vi "Main.vi"() -> ()   [LabVIEW 2013]
doc: "This template is for the Queued Message Handler design pattern.\n\nThe Event Handling Loop generates messages based on user interface actions.\n\nThe Message Handling Loop processes messages generated by the Event Handling Loop, or by other messages. The messages are string values, so new messages can be added easily to the Message Cases case structure in the Message Handling Loop. Each message cluster can also provide an optional value for Message Data, which is a variant that can be converted to whatever message-specific data is required."
uses:
  <vilib>/vision/Image Controls.llb/IMAQ Image.ctl
  Message Passing/MsgQ Loops enum.ctl
  Image Processing/Mask ROI FG Enum.ctl
  System Status/Status FG Enum.ctl
  Globals/Average Sector Data.vi
  controls/UI Data.ctl
  Message Queue/Message Queue.lvlib
  User Event - Stop/User Event - Stop.lvlib
  Image Processing/Image Processing.lvlib
  Common/State Machines/State Machine Lib.lvlib
  Message Passing/Main MsgQ.lvlib
  Common/GUI/GUI.lvlib
  <vilib>/rvi/interface/nirviReadWriteControl/nirviReadWriteControl.xnode
  FGs/FPGA_Reference.ctl
  FPGA Bitfiles/8-Tap8-bitCamera_FPGATarget_8-Tap8-bit_Serial_Server.lvbitx
  <vilib>/rvi/errors/niLvFpgaMergeErrorWithErrorCode.vi
  NiFpgaLv.dll
  <vilib>/rvi/errors/niLvFpgaAdjustHostInterfaceError.vi
panel:
  out "Analysis Ticks":u32
  out "Accumulate Ticks":u32
  out "FPGA Display Image":T1(plugin-control)
  out "Right Wingbeat Avg Graph":u8[](graph)
  in  "Start Serial Server":bool=TRUE
  out "Left Wingbeat Avg Graph":u8[](graph)
  in  "Stop Charts":bool
  in  "Wing ROIs":T2
  out "FPGA image info":T5={"Image Type"=0, "Unit"=enum."Undefined", "X Resolution"=2040, "Y Resolution"=1088, "X Step"=1.0, "Y Step"=1.0, "Image Name"="Image"} {"Image Type" items=["Grayscale (U8)", "Grayscale (I16)", "Grayscale (SGL)", "Complex (CSG)", "RGB (U32)", "HSL (U32)", "RGB (U64)", "Grayscale (U16)"]}
  in  "Stream?":bool
  out "FPGA Image":T1
  in  "Test Visual Response":bool
  in  "Test FPGA":bool
  out "Status Update":string="VI Stopped"
  in  "Define Mask":bool
  in  "Acquire Image":bool
  in  "Stop":bool
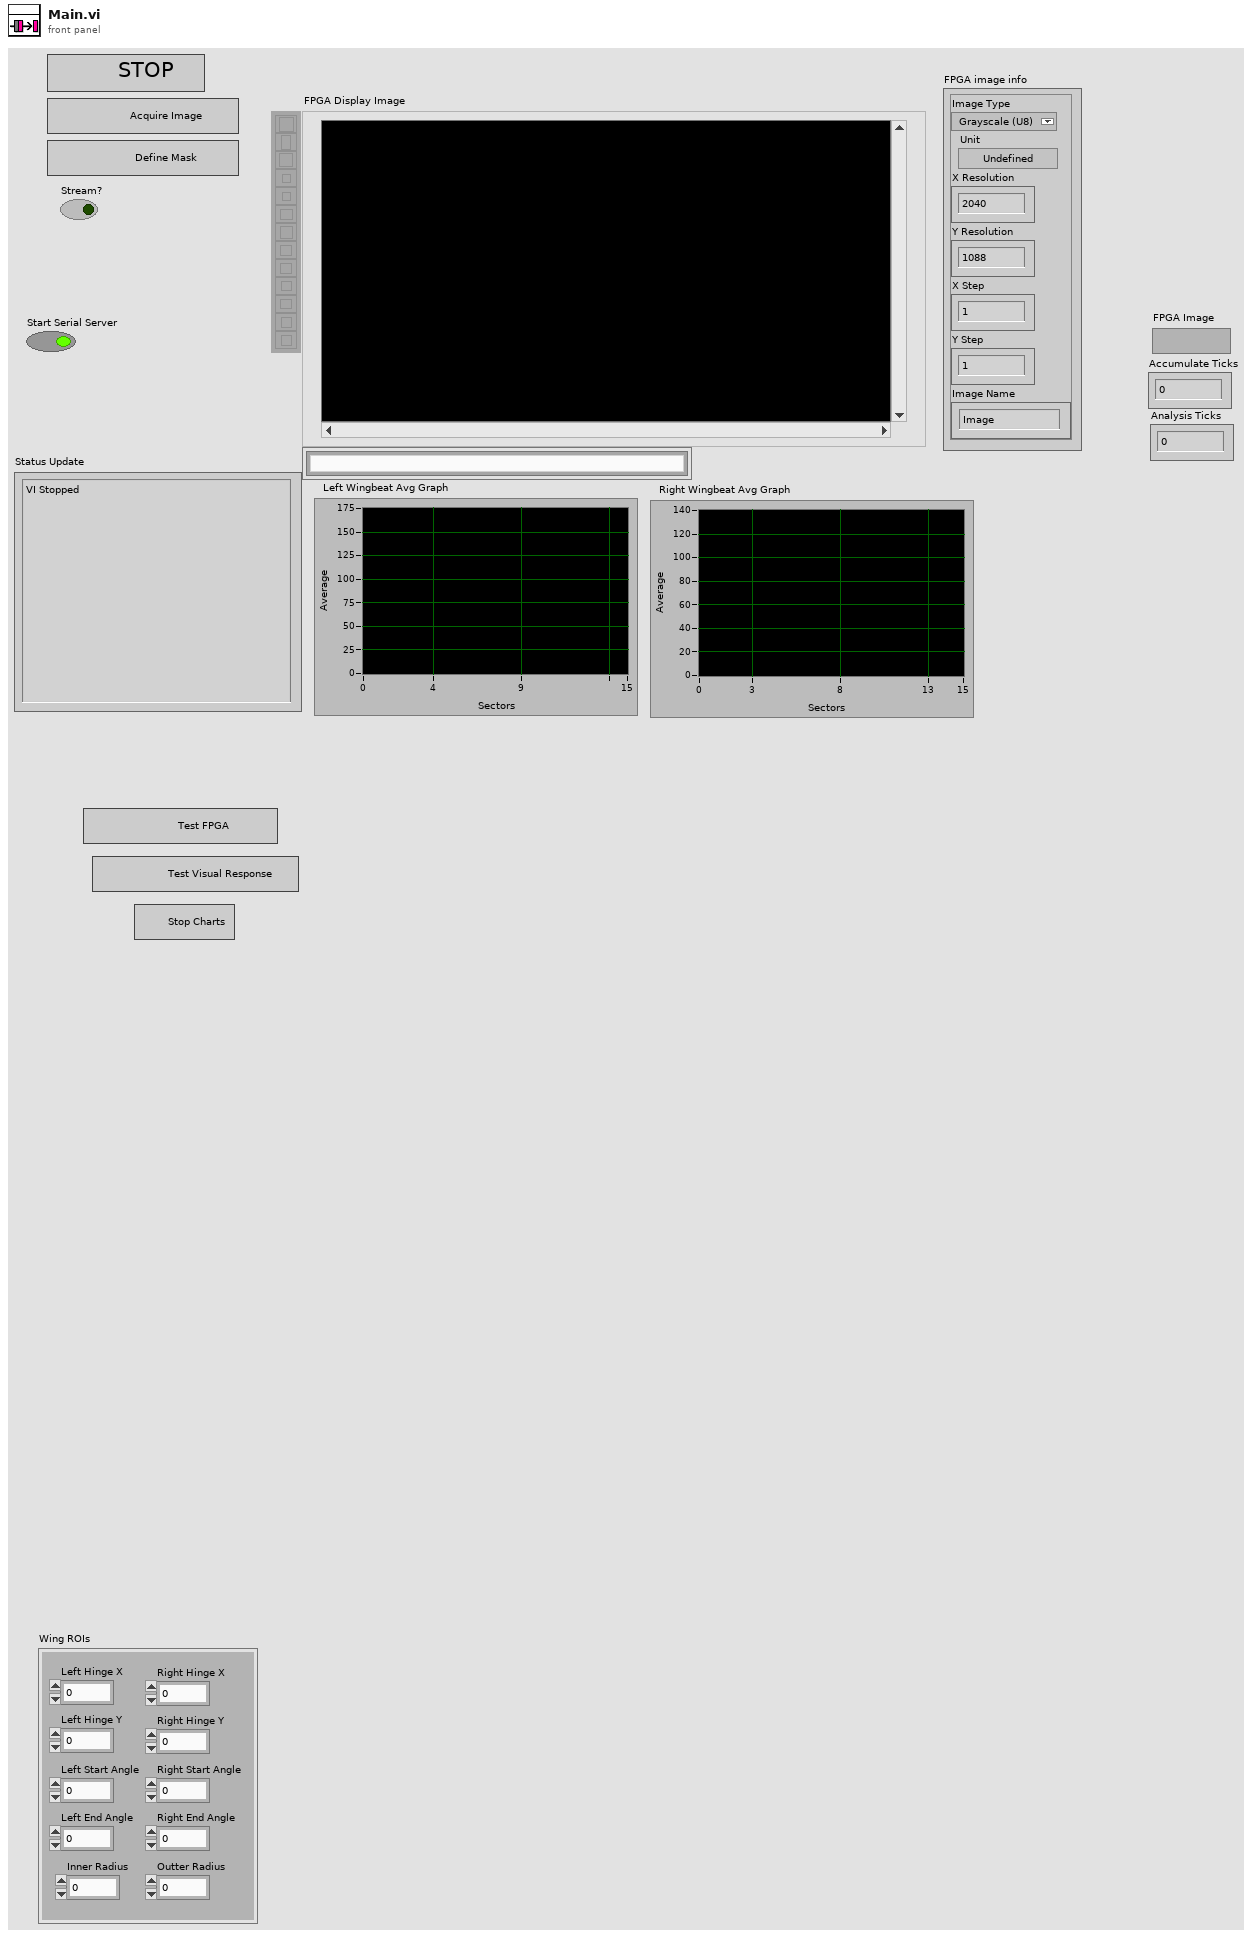
[diagram p1: front panel]
types:
  T1 = typedef "IMAQ Image.ctl" = refnum<image>
  T2 = cluster{"Left Hinge X":u16, "Left Hinge Y":u16, "Inner Radius":u16, "Outter Radius":u16, "Right Hinge X":u16, "Right Hinge Y":u16, "Right Start Angle":i16, "Right End Angle":i16, "Left Start Angle":i16, "Left End Angle":i16}
  T3 = typedef "Image Type" = u32
  T4 = typedef "Image Unit" = enum32{"Undefined", "Angström", "Micrometer", "Millimeter", "Centimeter", "Meter", "Kilometer", "Microinch", "Inch", "Feet", "Nautical miles", "Standard miles", "Steps"}
  T5 = cluster{"Image Type":T3, "Unit":T4, "X Resolution":i32, "Y Resolution":i32, "X Step":sgl, "Y Step":sgl, "Image Name":string}
  T6 = typedef "State Machine Lib.lvlib/STATE cluster.ctl" = cluster{"State":string, "Parameters":variant}
  T7 = typedef "Main MsgQ.lvlib/MsgQ Loops enum.ctl" = enum16{"User Interface", "Image Acq"}
  T8 = typedef "Status FG Enum.ctl" = enum16{"Reset", "Read", "Write"}
  T9 = typedef "Mask ROI FG Enum.ctl" = enum16{"Read", "Write"}
  T10 = typedef "FPGA_Reference.ctl" = refnum<k20>
  T11 = typedef "Mask ROI Cluster.ctl" = cluster{"left annulus":T12, "right annulus":T12, "Threshold Range":cluster{"Lower value":dbl, "Upper value":dbl}, "[Avg BG]":u8[], "Number of Sectors":u8, "Left ROI":T13, "Right ROI":T13, "Left Start Angle Duty Cycle":fxp<+,8,0>, "Left End Angle Duty Cycle":fxp<+,8,0>, "Right End Angle Duty Cycle":fxp<+,8,0>, "Right Start Angle Duty Cycle":fxp<+,8,0>, "[Sector ROIs]":T13[]}
  T12 = typedef "IMAQ Circle" = cluster{"Center X":i32, "Center Y":i32, "Inner Radius":i32, "Outer Radius":i32, "Start Angle":dbl, "End Angle":dbl}
  T13 = typedef "ROI Descriptor" = cluster{"Global Rectangle":i32[], "Contours":cluster{"ID":enum32{"External", "Internal"}, "Type":u32, "Coordinates":i32[]}[]}
  T14 = typedef "UI Data.ctl" = cluster{"Boolean <Replace Me>":bool, "Initial Message":string, "Numeric <Replace Me>":dbl, "Acquire Image Ref":refnum<vi>, "Define Mask Ref":refnum<vi>, "Status Update Ref":refnum<vi>, "Stop Button Ref":refnum<vi>, "FPGA Image":T1, "Processed Image":T1, "Left Annulus":cluster{"Center X":i32, "Center Y":i32, "Inner Radius":i32, "Outer Radius":i32, "Start Angle":dbl, "End Angle":dbl}, "Right Annulus":cluster{"Center X":i32, "Center Y":i32, "Inner Radius":i32, "Outer Radius":i32, "Start Angle":dbl, "End Angle":dbl}}
  T15 = typedef "Message Queue.lvlib/All Message Queues.ctl" = cluster{"UI":refnum<queue>}
  T16 = cluster{"Center X":i32, "Center Y":i32, "Inner Radius":i32, "Outer Radius":i32, "Start Angle":dbl, "End Angle":dbl}
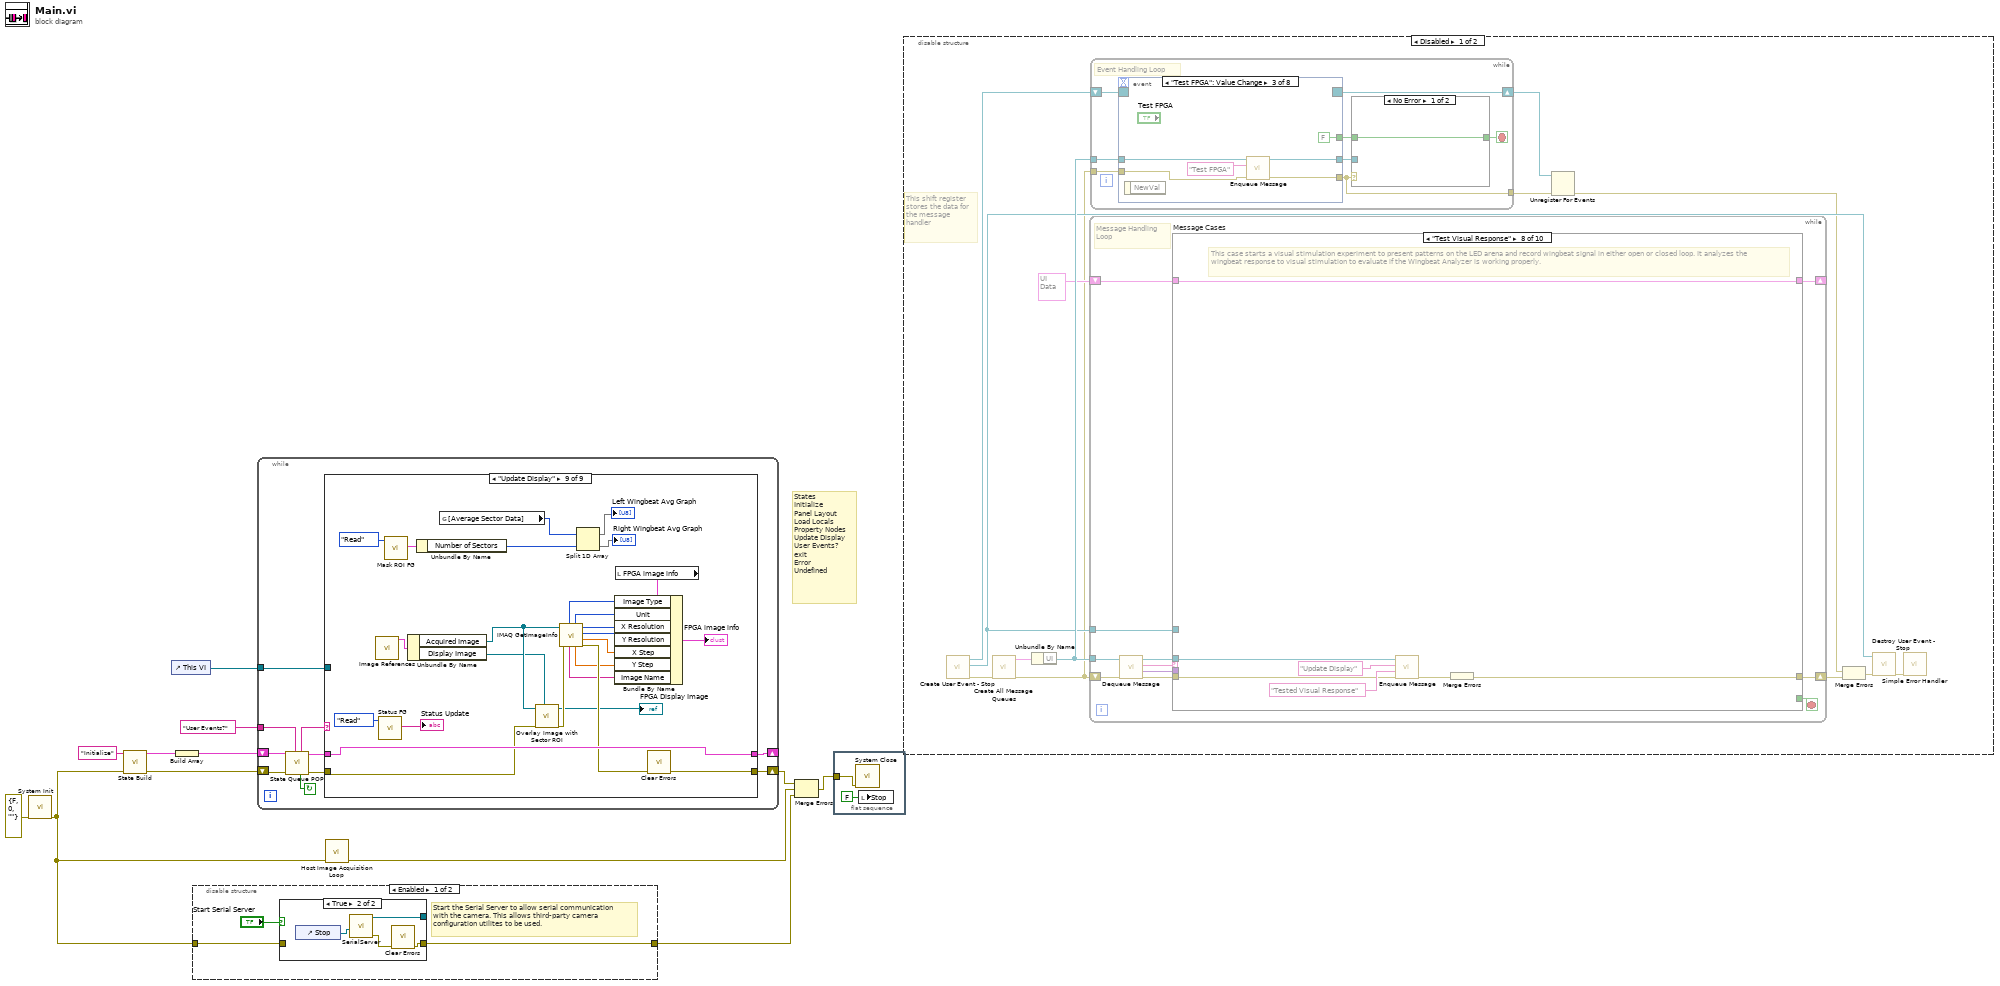
[diagram p0: block diagram]
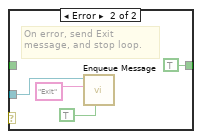
[diagram p4: hidden frame]
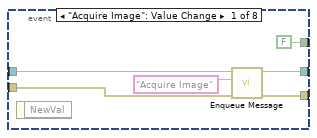
[diagram p5: hidden frame]
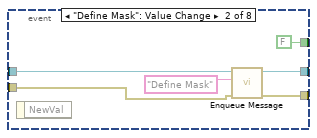
[diagram p6: hidden frame]
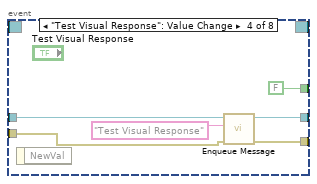
[diagram p7: hidden frame]
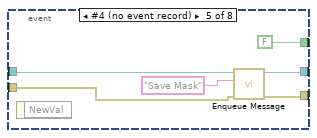
[diagram p8: hidden frame]
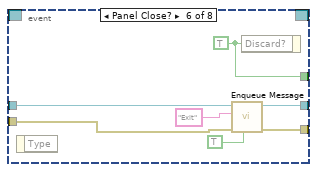
[diagram p9: hidden frame]
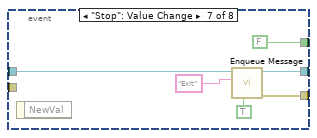
[diagram p10: hidden frame]
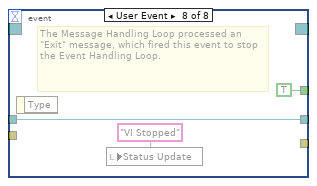
[diagram p11: hidden frame]
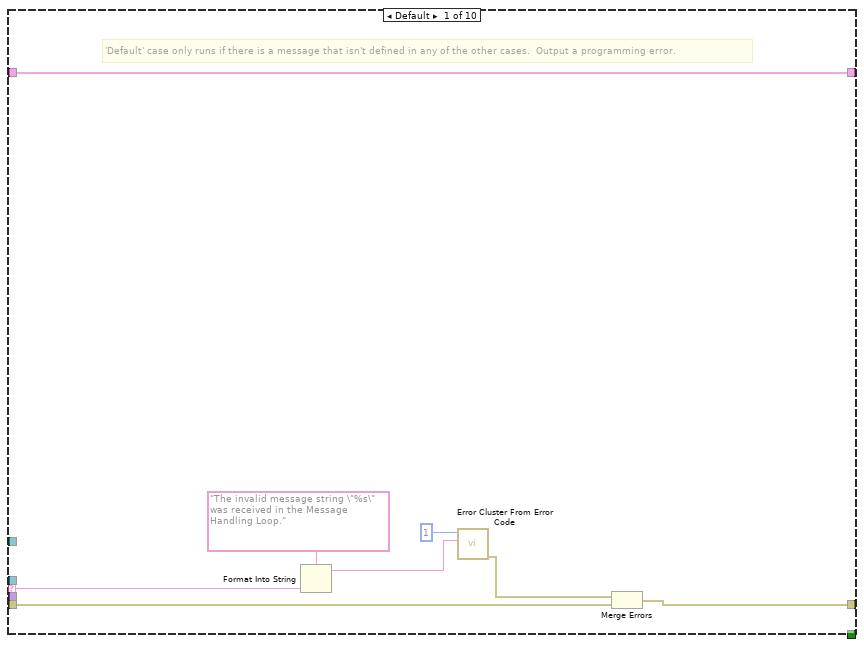
[diagram p12: hidden frame]
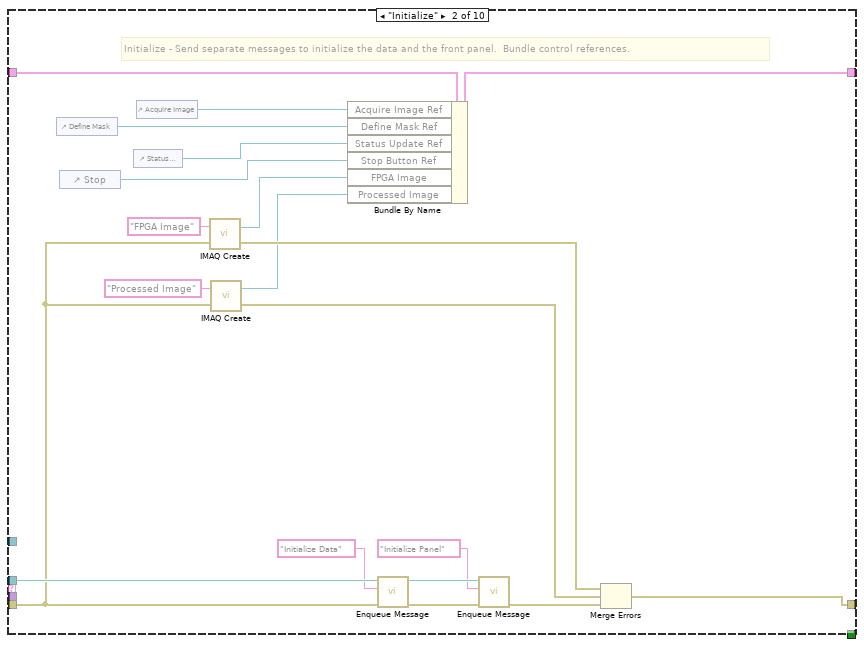
[diagram p13: hidden frame]
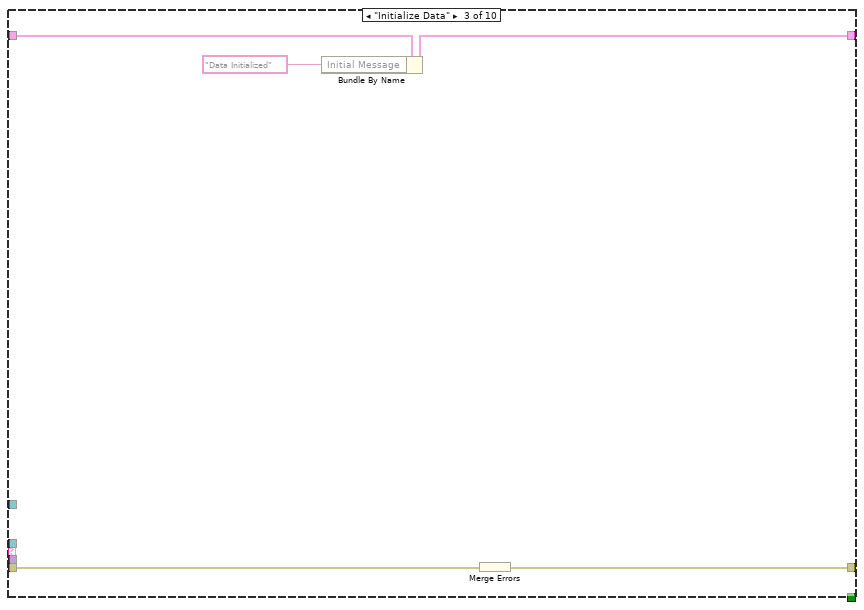
[diagram p14: hidden frame]
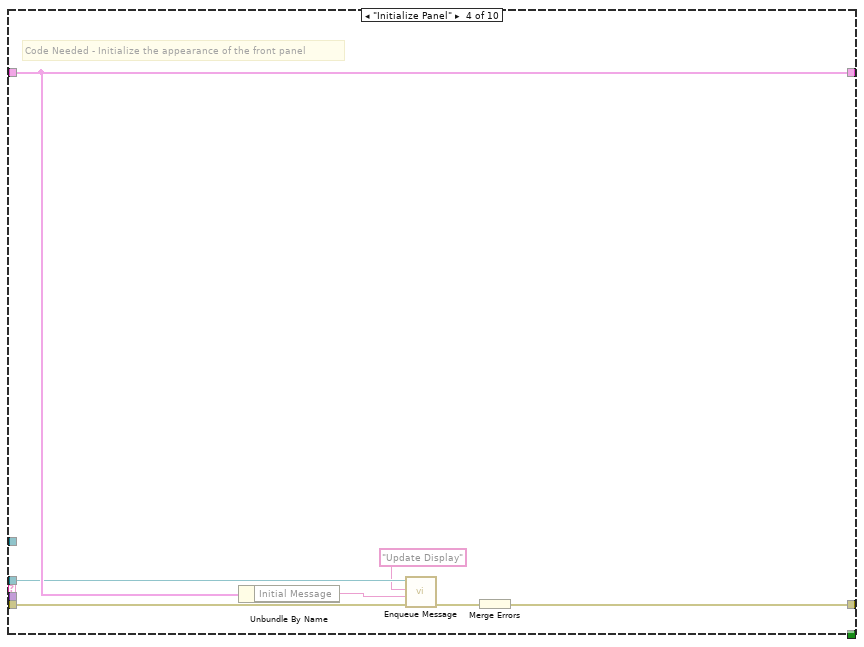
[diagram p15: hidden frame]
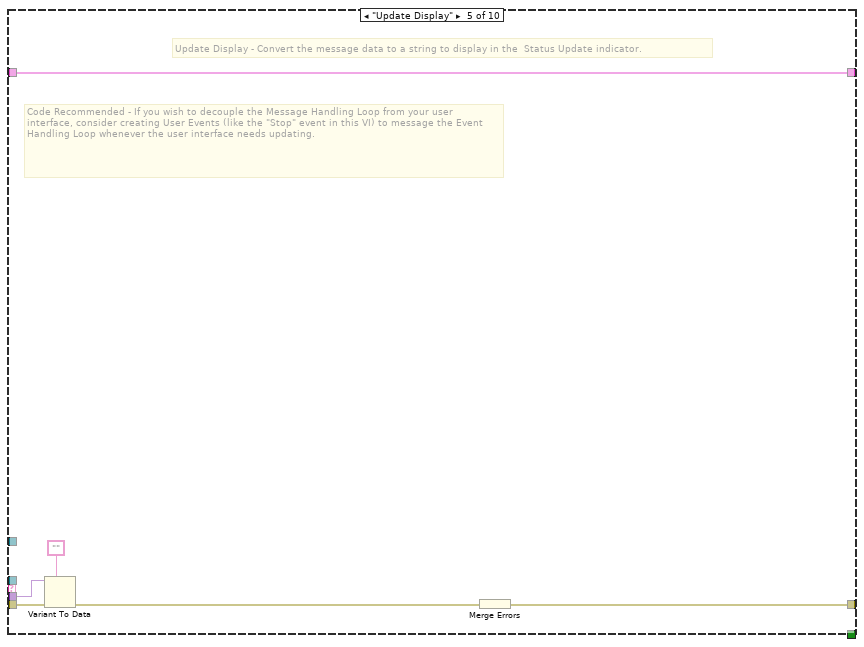
[diagram p16: hidden frame]
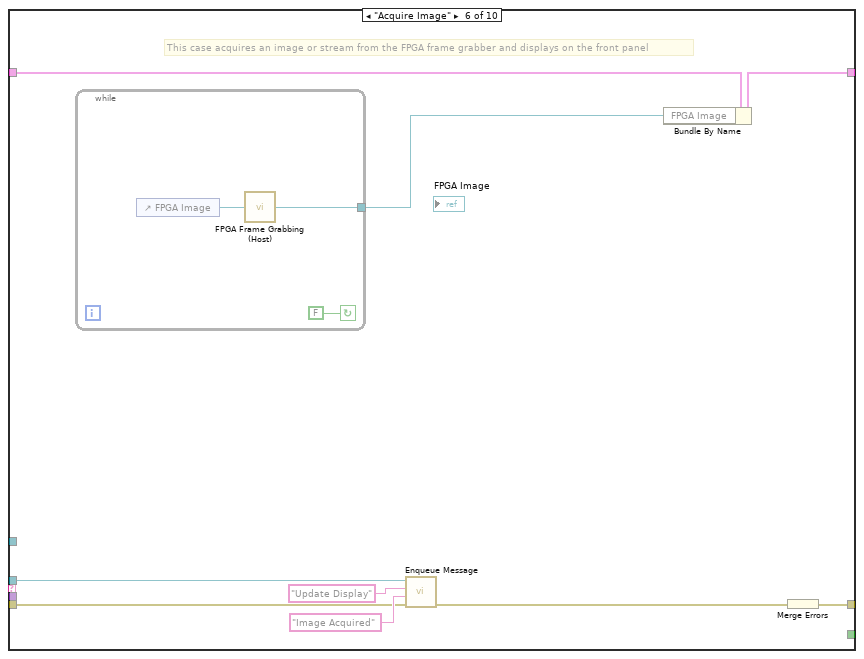
[diagram p17: hidden frame]
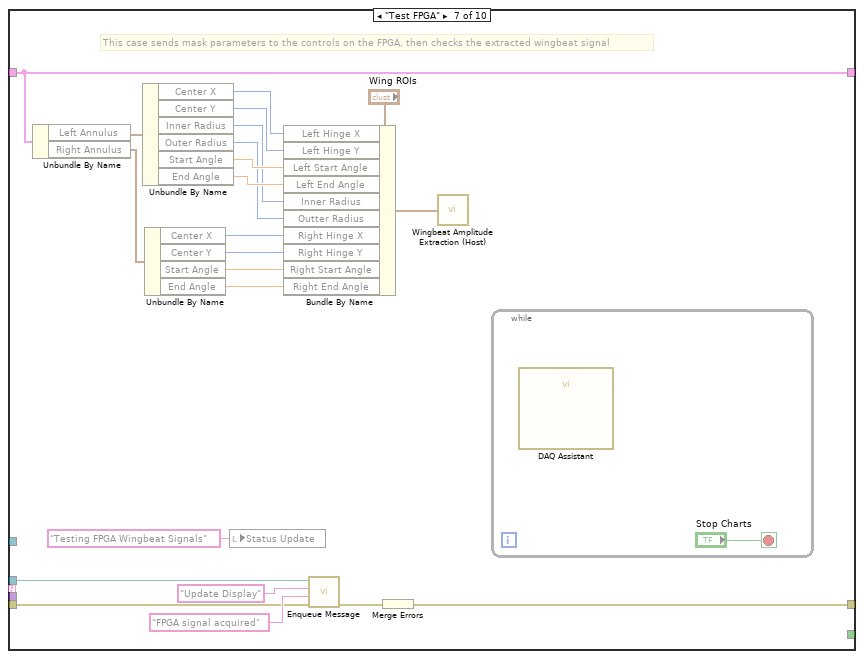
[diagram p18: hidden frame]
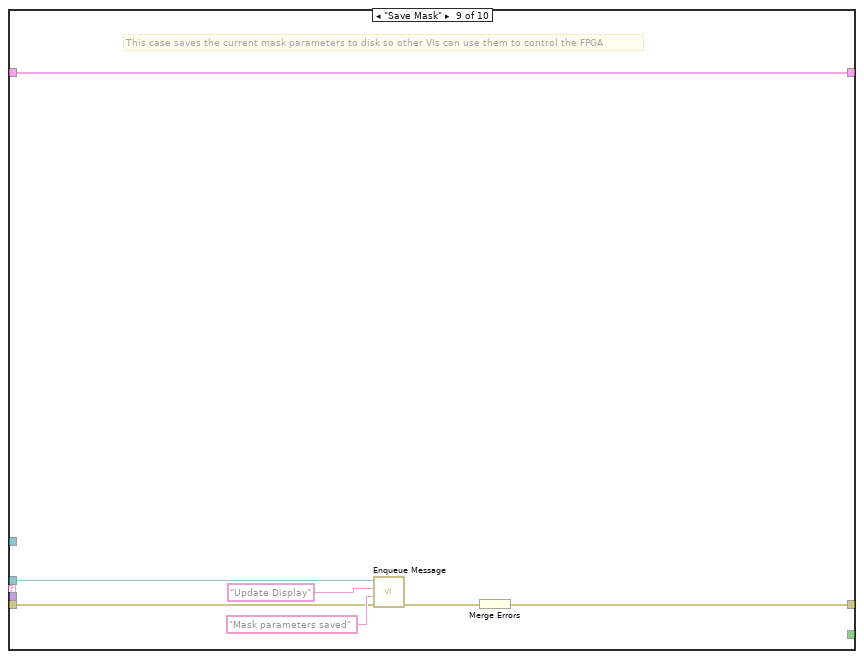
[diagram p19: hidden frame]
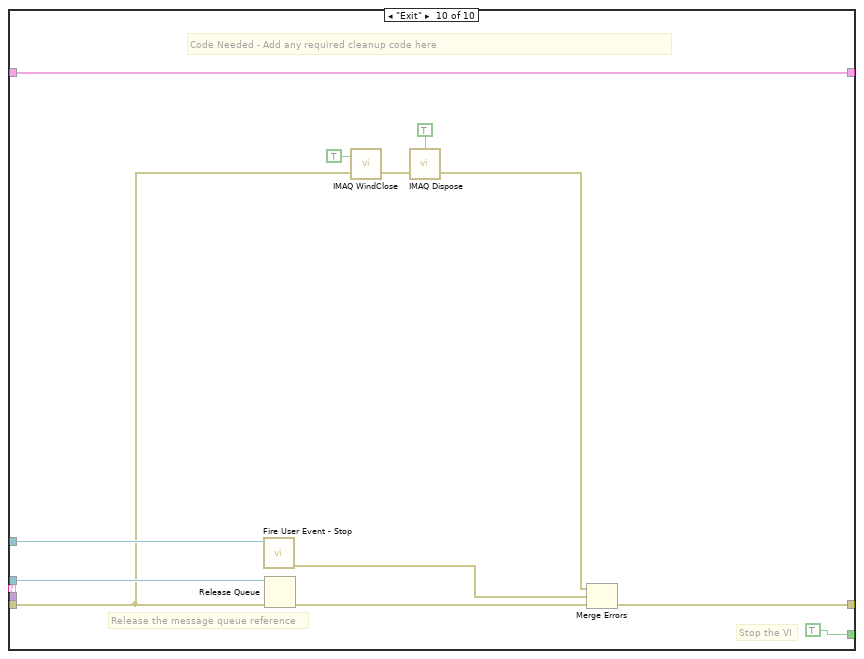
[diagram p20: hidden frame]
diagram:
  # "States\nInitialize\nPanel Layout\nLoad Locals\nProperty Nodes\nUpdate Display\nUser Events?\nexit\nError\nUndefined"
  n1 = call "System Init.vi"("error in (no error)"=errorcluster {"status"=FALSE, "code"=0, "source"=""}) -> ("error out"=w11:errorcluster)  [unwired: 10 in]
  n2 = call "State Build.vi"("error in (no error)"=w11, "State"="Initialize") -> ("error out"=w7:errorcluster, "State Out"=w9:T6)  [unwired: 8 in]
  n3 = control-ref of="This VI"() -> (w5:refnum<vi>)
  n4 = Build Array(w9) -> (w8:T6[])
  n5 = disable-structure shown="Enabled" {
    disable-tunnel: w11 -> [w14 _]
    disable-tunnel: [w13 _] -> w1
    frame Enabled {
      # "Start the Serial Server to allow serial communication\nwith the camera. This allows third-party camera\nconfiguration utilites to be used."
      n6 = case shown="True" "Start Serial Server" {
        tunnel: [_ w20] -> _
        tunnel: w14 -> [w16 _]
        tunnel: [w16 w18] -> w13
        frame False {
        }
        frame True {
          n7 = control-ref of="Stop"() -> (w19:refnum<vi>)
          n8 = call "SerialServer.vi"("Stop Refnum"=w19) -> ("error out"=w17:errorcluster, "FPGA VI Reference Out"=w20:refnum<k20>)  [unwired: 5 in]
          n9 = call <vilib>:"Clear Errors.vi"("error in (no error)"=w17) -> ("error out"=w18:errorcluster)  [unwired: 6 in]
        }
      }
    }
    frame Disabled {
    }
  }
  n10 = while {
    shift-right: [w24] -> _
    shift-left: w8 -> [w30]
    shift-right: [w22] -> w4
    shift-left: w7 -> [w29]
    tunnel: "User Events?" ("State") -> [w27]
    tunnel: w5 -> [w25]
    stop <- w28 continue-if-true
    n11 = call "State Queue POP.vi"("Default state"=w27, "error in (no error)"=w29, "State que in"=w30) -> ("error out"=w21:errorcluster, "State que out"=w23:T6[], "Not Exit?"=w28:bool, "State case out"=w26:string)  [unwired: 4 in, 1 out]
    n12 = case shown="\"Update Display\"" w26 {
      tunnel: w25 -> [_ _ w41 _ _ _ _ _ _]
      tunnel: [w32 w33 w38 w44 w46 w51 w55 w87 w114] -> w24
      tunnel: w23 -> [w32 w36 w38 w44 w46 w51 w54 _ w114]
      tunnel: [w31 w34 w39 w42 w45 w49 w53 w86 w112] -> w22
      tunnel: w21 -> [w31 w35 w40 w42 w45 w50 w52 w88 w96]
      frame Default {
      }
      frame "Initialize" {
        n13 = call "State Queue PUSH multiple states no parameters.vi"("States to queue"=string[] ["Panel Layout", "Load Locals", "Property Nodes", "Update Display"], "error in (no error)"=w35, "State que in"=w36) -> ("error out"=w34:errorcluster, "State que out"=w33:T6[])  [unwired: 7 in]
      }
      frame "Panel Layout" {
        # "Reset origin to 0,0"
        n14 = call "Reset all pane origins.vi"("error in (no error"=w40, "Vi Ref In"=w41) -> ("error out"=w39:errorcluster)  [unwired: 8 in, 1 out]
      }
      frame "Load Locals" {
        n15 = local write "Stream?"(FALSE ("Stream?")) -> ()
      }
      frame "Property Nodes" {
      }
      frame "Define Mask" {
        n16 = call "Image References.vi"() -> ("Images"=w48:cluster{"Acquired Image":T1, "Display Image":T1})  [unwired: 10 in, 1 out]
        n17 = Unbundle By Name(w48) -> ("Acquired Image"=w47:T1)
        n18 = call "Define Mask.vi"("error in (no error)"=w50, "FPGA Image"=w47) -> ("error out"=w49:errorcluster)  [unwired: 9 in]
      }
      frame "User Events?" {
        n19 = event shown="[4] \"Stop\": Value Change" {
          selector: _ -> [_ _ _ _ _]
          dyn-events: _ -> [_ _ _ _ _]
          timeout: 200 -> [_ _ _ _ _]
          tunnel: [w58 w68 w71 w78 w81] -> w55
          tunnel: w54 -> [w59 w68 w71 w80 w84]
          tunnel: [w60 w65 w72 w77 w82] -> w53
          tunnel: w52 -> [w61 w66 w73 w79 w83]
          event Timeout {
            n20 = event-data() -> ()  [unwired: 1 in, 3 out]
            n21 = disable-structure shown="Enabled" {
              frame Disabled {
                n22 = call "FPGA Reference FG.vi"() -> ("FPGA VI Reference Out"=w64:T10)  [unwired: 11 in]
                n23 = xnode "Read/Write Control"("FPGA VI Reference In"=w64) -> ("Accumulate Ticks"=→"Accumulate Ticks", "Analysis Ticks"=→"Analysis Ticks":u32)  [unwired: 1 in, 2 out]
              }
              frame Enabled {
              }
            }
            n24 = call "State Queue PUSH.vi"("State case"="Update Display", "error in (no error)"=w61, "State que in"=w59) -> ("error out"=w60:errorcluster, "State que out"=w58:T6[])  [unwired: 7 in]
          }
          event "Acquire Image": Value Change {
            n25 = event-data() -> ()  [unwired: 1 in, 6 out]
            n26 = call "Send MsgQ.vi"("error in (no error)"=w66, "Message String"="Acquire Single Image", "Send to MsgQ"=MsgQ_Loops_enum."Image Acq") -> ("error out"=w65:errorcluster)  [unwired: 8 in]
          }
          event "Stream?": Value Change {
            n27 = event-data() -> ("NewVal"=w70:bool)  [unwired: 1 in, 5 out]
            n28 = call "Send MsgQ.vi"("error in (no error)"=w73, "Data In"=w70, "Message String"="Stream Image", "Send to MsgQ"=MsgQ_Loops_enum."Image Acq") -> ("error out"=w72:errorcluster)  [unwired: 7 in]
          }
          event "Define Mask": Value Change {
            n29 = event-data() -> ()  [unwired: 1 in, 6 out]
            n30 = call "State Queue PUSH.vi"("State case"="Define Mask", "error in (no error)"=w79, "State que in"=w80) -> ("error out"=w77:errorcluster, "State que out"=w78:T6[])  [unwired: 7 in]
          }
          event "Stop": Value Change {
            n31 = event-data() -> ()  [unwired: 1 in, 6 out]
            n32 = call "State Queue PUSH.vi"("State case"="exit", "error in (no error)"=w83, "State que in"=w84) -> ("error out"=w82:errorcluster, "State que out"=w81:T6[])  [unwired: 7 in]
          }
        }
      }
      frame "exit" {
        n33 = call "Broadcast Exit.vi"("error in"=w88) -> ("error out"=w86:errorcluster)  [unwired: 10 in]
        n34 = call "Queue EXIT state.vi"() -> ("Exit State Q"=w87:T6[])  [unwired: 1 in]
      }
      frame "Update Display" {
        n35 = call "Image References.vi"() -> ("Images"=w91:cluster{"Acquired Image":T1, "Display Image":T1})  [unwired: 10 in, 1 out]
        n36 = call "Status FG.vi"("Operation"=Status_FG_Enum."Read") -> ("Status Out"=→"Status Update":string)  [unwired: 9 in, 1 out]
        n37 = call "Mask ROI FG.vi"("Operation"=Mask_ROI_FG_Enum."Read") -> ("Mask ROI Out"=w109:T11)  [unwired: 9 in, 1 out]
        n38 = Unbundle By Name(w91) -> ("Acquired Image"=w90:T1, "Display Image"=w89:T1)
        n39 = Unbundle By Name(w109) -> ("Number of Sectors"=w106:u8)
        n40 = global read "Average Sector Data.vi" "[Average Sector Data]"() -> (w111:u8[])
        n41 = call "Overlay Image with Sector ROI.vi"("FPGA Display Image In"=w89, "error in"=w96, "FPGA Image"=w90) -> ("error out"=w95:errorcluster, "FPGA Display Image Out"=→"FPGA Display Image":T1)  [unwired: 7 in]
        n42 = call "IMAQ GetImageInfo"("error in (no error)"=w95, "Image"=w90) -> ("error out"=w113:errorcluster, "X Step"=w101:sgl, "Y Resolution"=w100:i32, "X Resolution"=w99:i32, "Y Step"=w102:sgl, "Unit"=w98:T4, "Image Name"=w103:string, "Image Type"=w97:T3)  [unwired: 2 in]
        n43 = Split 1D Array(array=w111, index=w106) -> (first subarray=→"Left Wingbeat Avg Graph":u8[], second subarray=→"Right Wingbeat Avg Graph":u8[])
        n44 = local read "FPGA image info"() -> (w105:T5)
        n45 = Bundle By Name(cluster=w105, "Image Type"=w97, "Unit"=w98, "X Resolution"=w99, "Y Resolution"=w100, "X Step"=w101, "Y Step"=w102, "Image Name"=w103) -> (→"FPGA image info":T5)
        n46 = call <vilib>:"Clear Errors.vi"("error in (no error)"=w113) -> ("error out"=w112:errorcluster)  [unwired: 6 in]
      }
    }
  }
  n47 = call "Host Image Acquisition Loop.vi"("error in"=w11) -> ("error out"=w3:errorcluster)  [unwired: 10 in]
  n48 = Merge Errors(w4, w3, w1) -> (w2:errorcluster)
  n49 = flat-sequence {
    tunnel: w2 -> [w116]
    frame #0 {
      n50 = call "System Close.vi"("error in (no error)"=w116) -> ()  [unwired: 10 in, 1 out]
      n51 = local write "Stop"(FALSE ("Stop")) -> ()
    }
  }
  n52 = disable-structure shown="Disabled" {
    frame Disabled {
      # "This shift register\nstores the data for the message handler"
      n53 = call "Create User Event - Stop.vi"() -> ("error out"=w125:errorcluster, "User Event - Stop"=w122:refnum<user-event>, "Stop Event Registration Refnum"=w126:refnum<event-registration>)  [unwired: 9 in]
      n54 = call "Create All Message Queues.vi"("error in (no error)"=w125) -> ("error out"=w117:errorcluster, "Message Queues out"=w129:T15)  [unwired: 9 in]
      n55 = Unbundle By Name(w129) -> ("UI"=w127:refnum<queue>)
      n56 = while {
        tunnel: w127 -> [w189]
        shift-right: [w198] -> _
        shift-left: T14 {"Boolean <Replace Me>"=TRUE, "Initial Message"="", "Numeric <Replace Me>"=0.0, "Acquire Image Ref"=refnum, "Define Mask Ref"=refnum, "Status Update Ref"=refnum, "Stop Button Ref"=refnum, "FPGA Image"=refnum, "Processed Image"=refnum, "Left Annulus"={"Center X"=0, "Center Y"=0, "Inner Radius"=0, "Outer Radius"=0, "Start Angle"=0.0, "End Angle"=0.0}, "Right Annulus"={"Center X"=0, "Center Y"=0, "Inner Radius"=0, "Outer Radius"=0, "Start Angle"=0.0, "End Angle"=0.0}} ("Data Cluster") -> [w199]
        tunnel: w122 -> [w195]
        shift-right: [w196] -> w128
        shift-left: w117 -> [w194]
        stop <- w197 stop-if-true
        # "Message Handling Loop"
        n57 = call "Dequeue Message.vi"("error in (no error)"=w194, "Message Queue"=w189) -> ("error out"=w193:errorcluster, "Message Data"=w191:variant, "Message"=w192:string, "dup Message Queue"=w190:refnum<queue>)  [unwired: 6 in]
        n58 = case "Message Cases" shown="\"Test Visual Response\"" w192 {
          selector: w192 -> [w205 _ _ _ _ _ _ _ _ _]
          tunnel: w190 -> [_ w225 _ w236 _ w253 w276 w284 w292 w308]
          tunnel: w193 -> [w202 w210 w232 w237 w244 w248 w277 w285 w290 w297]
          tunnel: [w200 w212 w228 w238 w245 w255 w275 w283 w295 w304] -> w196
          tunnel: w199 -> [w207 w222 w231 w239 w246 w250 w274 w289 w296 w307]
          tunnel: [w207 w221 w230 w239 w246 w249 w274 w289 w296 w307] -> w198
          tunnel: [_ _ _ _ _ _ _ _ _ TRUE] -> w197
          tunnel: w191 -> [_ _ _ _ w243 _ _ _ _ _]
          tunnel: w195 -> [_ _ _ _ _ _ _ _ _ w303]
          frame Default {
            # "'Default' case only runs if there is a message that isn't defined in any of the other cases.  Output a programming error."
            n59 = Format Into String(format string="The invalid message string \"%s\" was received in the Message Handling Loop." ("Unknown Message Error Text"), w205) -> (resulting string=w203:string)  [unwired: 2 in, 1 out]
            n60 = call <vilib>:"Error Cluster From Error Code.vi"("error message (\"\")"=w203, "error code (0)"=1) -> ("error out"=w201:errorcluster)  [unwired: 7 in]
            n61 = Merge Errors(w201, w202) -> (w200:errorcluster)
          }
          frame "Initialize" {
            # "Initialize - Send separate messages to initialize the data and the front panel.  Bundle control references."
            n62 = control-ref of="Define Mask"() -> (w219:refnum<vi>)
            n63 = control-ref of="Stop"() -> (w217:refnum<vi>)
            n64 = control-ref of="Status Update"() -> (w218:refnum<vi>)
            n65 = control-ref of="Acquire Image"() -> (w220:refnum<vi>)
            n66 = call "IMAQ Create"("Image Name"="FPGA Image", "error in (no error)"=w210) -> ("New Image"=w215:T1, "error out"=w211:errorcluster)  [unwired: 3 in]
            n67 = call "IMAQ Create"("Image Name"="Processed Image", "error in (no error)"=w210) -> ("New Image"=w208:T1, "error out"=w209:errorcluster)  [unwired: 3 in]
            n68 = Bundle By Name(cluster=w222, "Acquire Image Ref"=w220, "Define Mask Ref"=w219, "Status Update Ref"=w218, "Stop Button Ref"=w217, "FPGA Image"=w215, "Processed Image"=w208) -> (w221:T14)
            n69 = call "Enqueue Message.vi"("error in (no error)"=w210, "Message"="Initialize Data", "Message Queue"=w225) -> ("error out"=w227:errorcluster, "dup Message Queue"=w226:refnum<queue>)  [unwired: 7 in]
            n70 = call "Enqueue Message.vi"("error in (no error)"=w227, "Message"="Initialize Panel", "Message Queue"=w226) -> ("error out"=w213:errorcluster)  [unwired: 7 in, 1 out]
            n71 = Merge Errors(w211, w209, w213) -> (w212:errorcluster)
          }
          frame "Initialize Data" {
            n72 = Bundle By Name(cluster=w231, "Initial Message"="Data Initialized") -> (w230:T14)
            n73 = Merge Errors(w232) -> (w228:errorcluster)
          }
          frame "Initialize Panel" {
            # "Code Needed - Initialize the appearance of the front panel"
            n74 = Unbundle By Name(w239) -> ("Initial Message"=w233:string)
            n75 = call "Enqueue Message.vi"("error in (no error)"=w237, "Message Data"=w233, "Message"="Update Display", "Message Queue"=w236) -> ("error out"=w235:errorcluster)  [unwired: 6 in, 1 out]
            n76 = Merge Errors(w235) -> (w238:errorcluster)
          }
          frame "Update Display" {
            # "Code Recommended - If you wish to decouple the Message Handling Loop from your user interface, consider creating User Events (like the \"Stop\" event in this VI) to message the Event Handling Loop whenever the user interface needs updating."
            # "Update Display - Convert the message data to a string to display in the  Status Update indicator."
            n77 = Variant To Data(error in=w244, type="", Variant=w243) -> (data=w240:string, error out=w241:errorcluster)
            n78 = Merge Errors(w241) -> (w245:errorcluster)
          }
          frame "Acquire Image" {
            # "This case acquires an image or stream from the FPGA frame grabber and displays on the front panel"
            n79 = while {
              tunnel: [w258] -> w247
              stop <- FALSE continue-if-true
              n80 = control-ref of="FPGA Image"() -> (w257:refnum<vi>)
              n81 = call "FPGA Frame Grabbing (Host).vi"("Ctl Refnum"=w257) -> ("Image"=w258:T1)
            }
            n82 = call "Enqueue Message.vi"("error in (no error)"=w248, "Message Data"="Image Acquired" ("\"Do Something\" button pressed"), "Message"="Update Display", "Message Queue"=w253) -> ("error out"=w254:errorcluster)  [unwired: 6 in, 1 out]
            n83 = Bundle By Name(cluster=w250, "FPGA Image"=w247) -> (w249:T14)
            n84 = Merge Errors(w254) -> (w255:errorcluster)
          }
          frame "Test FPGA" {
            # "This case sends mask parameters to the controls on the FPGA, then checks the extracted wingbeat signal"
            n85 = Unbundle By Name(w274) -> ("Left Annulus"=w273:T16, "Right Annulus"=w272:T16)
            n86 = Unbundle By Name(w273) -> ("Center X"=w270:i32, "Center Y"=w269:i32, "Inner Radius"=w266:i32, "Outer Radius"=w265:i32, "Start Angle"=w268:dbl, "End Angle"=w267:dbl)
            n87 = Unbundle By Name(w272) -> ("Center X"=w264:i32, "Center Y"=w263:i32, "Start Angle"=w262:dbl, "End Angle"=w261:dbl)
            n88 = local write "Status Update"("Testing FPGA Wingbeat Signals" ("Status Update")) -> ()
            n89 = Bundle By Name(cluster="Wing ROIs", "Left Hinge X"=w270, "Left Hinge Y"=w269, "Left Start Angle"=w268, "Left End Angle"=w267, "Inner Radius"=w266, "Outter Radius"=w265, "Right Hinge X"=w264, "Right Hinge Y"=w263, "Right Start Angle"=w262, "Right End Angle"=w261) -> (w260:T2)
            n90 = call "Enqueue Message.vi"("error in (no error)"=w277, "Message Data"="FPGA signal acquired" ("\"Do Something\" button pressed"), "Message"="Update Display", "Message Queue"=w276) -> ("error out"=w280:errorcluster)  [unwired: 6 in, 1 out]
            n91 = Merge Errors(w280) -> (w275:errorcluster)
            n92 = call "Wingbeat Amplitude Extraction (Host).vi"("Wing ROIs"=w260) -> ()  [unwired: 1 in]
            n93 = while {
              stop <- "Stop Charts" stop-if-true
              n94 = call "DAQ Assistant"() -> ("data"=w281:dynamicdata)  [unwired: 17 in, 2 out]
            }
          }
          frame "Test Visual Response" {
            # "This case starts a visual stimulation experiment to present patterns on the LED arena and record wingbeat signal in either open or closed loop. It analyzes the wingbeat response to visual stimulation to evaluate if the Wingbeat Analyzer is working properly."
            n95 = call "Enqueue Message.vi"("error in (no error)"=w285, "Message Data"="Tested Visual Response" ("\"Do Something\" button pressed"), "Message"="Update Display", "Message Queue"=w284) -> ("error out"=w288:errorcluster)  [unwired: 6 in, 1 out]
            n96 = Merge Errors(w288) -> (w283:errorcluster)
          }
          frame "Save Mask" {
            # "This case saves the current mask parameters to disk so other VIs can use them to control the FPGA"
            n97 = call "Enqueue Message.vi"("error in (no error)"=w290, "Message Data"="Mask parameters saved" ("\"Do Something Else\" button pressed"), "Message"="Update Display", "Message Queue"=w292) -> ("error out"=w291:errorcluster)  [unwired: 6 in, 1 out]
            n98 = Merge Errors(w291) -> (w295:errorcluster)
          }
          frame "Exit" {
            # "Stop the VI"
            # "Release the message queue reference"
            # "Code Needed - Add any required cleanup code here"
            n99 = call "Fire User Event - Stop.vi"("User Event - Stop"=w303) -> ("error out"=w302:errorcluster)  [unwired: 10 in]
            n100 = Release Queue(queue=w308, error in (no error)=w297) -> (error out=w305:errorcluster)  [unwired: 1 in, 2 out]
            n101 = call "IMAQ WindClose"("Close All Windows (False)"=TRUE, "error in (no error)"=w297) -> ("error out"=w299:errorcluster)  [unwired: 4 in]
            n102 = call "IMAQ Dispose"("All Images? (No)"=TRUE, "error in (no error)"=w299) -> ("error out"=w298:errorcluster)  [unwired: 4 in]
            n103 = Merge Errors(w298, w302, w305) -> (w304:errorcluster)
          }
        }
      }
      n104 = while {
        tunnel: w127 -> [w137]
        tunnel: [w133] -> w120
        shift-right: [w131] -> w119
        shift-left: w126 -> [w132]
        tunnel: w117 -> [w130]
        stop <- w135 stop-if-true
        # "Event Handling Loop"
        n105 = event shown="[2] \"Test FPGA\": Value Change" {
          selector: w132 -> [_ _ _ _ _ _ _ _]
          dyn-events: [_ _ _ _ _ _ _ _] -> w131
          timeout: _ -> [_ _ _ _ _ _ _ _]
          tunnel: [FALSE ("Discard?") FALSE ("Discard?") FALSE ("Discard?") FALSE ("Discard?") FALSE ("Discard?") w179 FALSE ("Discard?") TRUE ("Discard?")] -> w136
          tunnel: w137 -> [w148 w154 w160 w165 w170 w178 w185 w188]
          tunnel: [w147 w152 w157 w162 w167 w177 w184 _] -> w133
          tunnel: [w146 w153 w156 w164 w169 w176 w182 w188] -> w134
          tunnel: w130 -> [w144 w150 w158 w161 w168 w173 _ _]
          event "Acquire Image": Value Change {
            n106 = event-data() -> ()  [unwired: 1 in, 1 out]
            n107 = call "Enqueue Message.vi"("error in (no error)"=w144, "Message"="Acquire Image", "Message Queue"=w148) -> ("error out"=w147:errorcluster, "dup Message Queue"=w146:refnum<queue>)  [unwired: 7 in]
          }
          event "Define Mask": Value Change {
            n108 = event-data() -> ()  [unwired: 1 in, 1 out]
            n109 = call "Enqueue Message.vi"("error in (no error)"=w150, "Message"="Define Mask", "Message Queue"=w154) -> ("error out"=w152:errorcluster, "dup Message Queue"=w153:refnum<queue>)  [unwired: 7 in]
          }
          event "Test FPGA": Value Change {
            n110 = event-data() -> ()  [unwired: 1 in, 1 out]
            n111 = call "Enqueue Message.vi"("error in (no error)"=w158, "Message"="Test FPGA", "Message Queue"=w160) -> ("error out"=w157:errorcluster, "dup Message Queue"=w156:refnum<queue>)  [unwired: 7 in]
          }
          event "Test Visual Response": Value Change {
            n112 = event-data() -> ()  [unwired: 1 in, 1 out]
            n113 = call "Enqueue Message.vi"("error in (no error)"=w161, "Message"="Test Visual Response", "Message Queue"=w165) -> ("error out"=w162:errorcluster, "dup Message Queue"=w164:refnum<queue>)  [unwired: 7 in]
          }
          event #4 (no event record) {
            n114 = event-data() -> ()  [unwired: 1 in, 1 out]
            n115 = call "Enqueue Message.vi"("error in (no error)"=w168, "Message"="Save Mask", "Message Queue"=w170) -> ("error out"=w167:errorcluster, "dup Message Queue"=w169:refnum<queue>)  [unwired: 7 in]
          }
          event Panel Close? {
            w179 = TRUE ("Discard?")
            n116 = event-data() -> ()  [unwired: 1 in, 1 out]
            n117 = call "Enqueue Message.vi"("Priority Message? (F)"=TRUE, "error in (no error)"=w173, "Message"="Exit", "Message Queue"=w178) -> ("error out"=w177:errorcluster, "dup Message Queue"=w176:refnum<queue>)  [unwired: 6 in]
            n118 = event-data("Discard?"=w179) -> ()  [unwired: 1 in, 1 out]
          }
          event "Stop": Value Change {
            n119 = event-data() -> ()  [unwired: 1 in, 1 out]
            n120 = call "Enqueue Message.vi"("Priority Message? (F)"=TRUE, "Message"="Exit", "Message Queue"=w185) -> ("error out"=w184:errorcluster, "dup Message Queue"=w182:refnum<queue>)  [unwired: 7 in]
          }
          event User Event {
            # "The Message Handling Loop processed an \"Exit\" message, which fired this event to stop the Event Handling Loop."
            n121 = event-data() -> ()  [unwired: 1 in, 1 out]
            n122 = local write "Status Update"("VI Stopped" ("VI Stopped")) -> ()
          }
        }
        n123 = case shown="No Error" w133 {
          tunnel: [w138 TRUE ("Discard?")] -> w135
          tunnel: w136 -> [w138 _]
          tunnel: w134 -> [_ w141]
          frame No Error {
          }
          frame Error {
            # "On error, send Exit message, and stop loop."
            n124 = call "Enqueue Message.vi"("Priority Message? (F)"=TRUE, "Message"="Exit", "Message Queue"=w141) -> ()  [unwired: 7 in, 2 out]
          }
        }
      }
      n125 = Unregister For Events(event registration refnum=w119, error in=w120) -> (error out=w121:errorcluster)
      n126 = Merge Errors(w121, w128) -> (w123:errorcluster)
      n127 = call "Destroy User Event - Stop.vi"("error in (no error)"=w123, "User Event - Stop"=w122) -> ("error out"=w124:errorcluster)  [unwired: 9 in]
      n128 = call <vilib>:"Simple Error Handler.vi"("error in (no error)"=w124) -> ()  [unwired: 4 in, 5 out]
    }
    frame Enabled {
    }
  }
